vi "cm2nm_rotate_about_origin.vi"(1 "Theta(deg)":dbl, 2 "In":cluster{"X":dbl, "Y":dbl, "Z":dbl}[](array[cluster])) -> (0 "Rotated":cluster{"X":dbl, "Y":dbl, "Z":dbl}[](array[cluster]))   [LabVIEW 2011]
doc: "rotate points about the origin by Theta (in degress)"
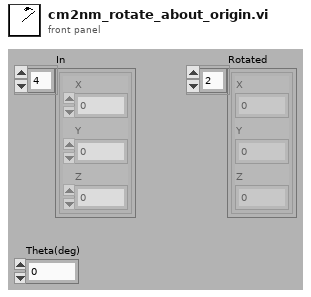
[diagram p1: front panel]
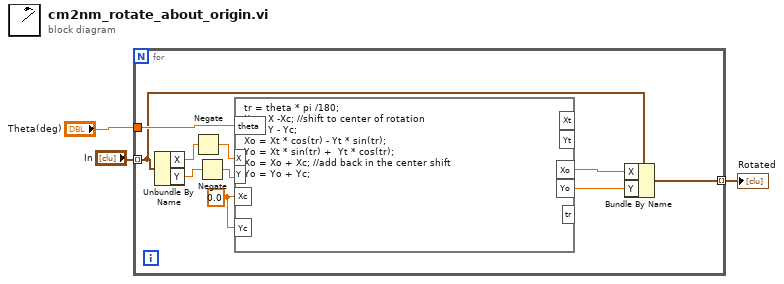
[diagram p0: block diagram]
diagram:
  n1 = for {
    tunnel: "In" -> [w11] mode=indexing
    tunnel: "Theta(deg)" -> [w12]
    tunnel: [w8] -> w3 mode=indexing
    w13 = 0.0 ("input variable")
    n2 = Unbundle By Name(w11) -> ("X"=w7:dbl, "Y"=w4:dbl)
    n3 = Negate(x=w7) -> (-x=w6:dbl)
    n4 = Negate(x=w4) -> (-x=w5:dbl)
    n5 = formula code="tr = theta * pi /180;\nXt = X -Xc; //shift to center of rotation\nYt = Y - Yc;\nXo = Xt * cos(tr) - Yt * sin(tr);\nYo = Xt * sin(tr) +  Yt * cos(tr);\nXo = Xo + Xc; //add back in the center shift\nYo = Yo + Yc;"("theta"=w12, "X"=w6, "Y"=w5, "Xc"=w13, "Yc"=w13) -> ("Xo"=w10:dbl, "Yo"=w9:dbl)  [unwired: 3 out]
    n6 = Bundle By Name(cluster=w11, "X"=w10, "Y"=w9) -> (w8:cluster{"X":dbl, "Y":dbl, "Z":dbl})
  }
  "Rotated" <- w3
